vi "日志、报警信息存储 (子VI).vi"() -> ()   [LabVIEW 2016, in "德润DR803F超标留样.lvlib"]
panel:
  out "仪器状态":T1 {"门状态" items=["关闭", "打开"]; "采样模式" items=["定时留样"=1, "时间等比"=2, "同步留样"=3, "外控留样"=4, "超标留样"=5]; "工作进程" items=["清洗管路初始化", "采样瓶位置初始化", "采样瓶排空", "清洗管下降", "采样瓶清洗", "清洗管上升", "外置泵延时", "管路润洗", "进样1", "进样2", "排空管路", "采样瓶位置调整", "待机"]; "仪器时间" format="%<%Y/%m/%d %H:%M:%S>T"; "工作状态" items=["停止", "运行"]}
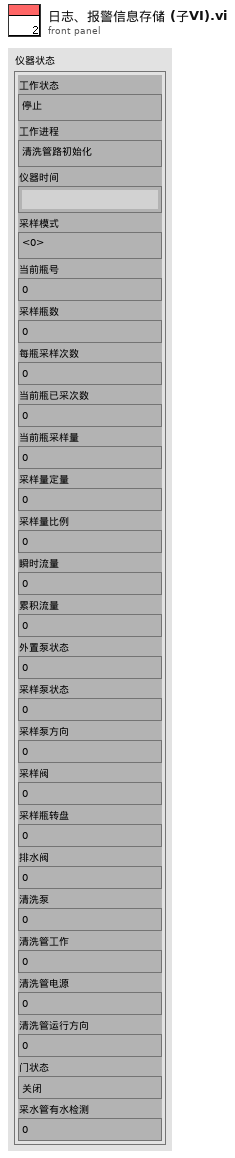
[diagram p1: front panel]
types:
  T1 = cluster{"工作状态":u16, "工作进程":u16, "仪器时间":timestamp, "采样模式":u16, "当前瓶号":dbl, "采样瓶数":dbl, "每瓶采样次数":dbl, "当前瓶已采次数":dbl, "当前瓶采样量":dbl, "采样量定量":dbl, "采样量比例":dbl, "瞬时流量":dbl, "累积流量":dbl, "外置泵状态":dbl, "采样泵状态":dbl, "采样泵方向":dbl, "采样阀":dbl, "采样瓶转盘":dbl, "排水阀":dbl, "清洗泵":dbl, "清洗管工作":dbl, "清洗管电源":dbl, "清洗管运行方向":dbl, "门状态":u16, "采水管有水检测":dbl}
  T2 = cluster{"时间标识":timestamp, "设备":string, "日志信息":string, "流程参数":string}
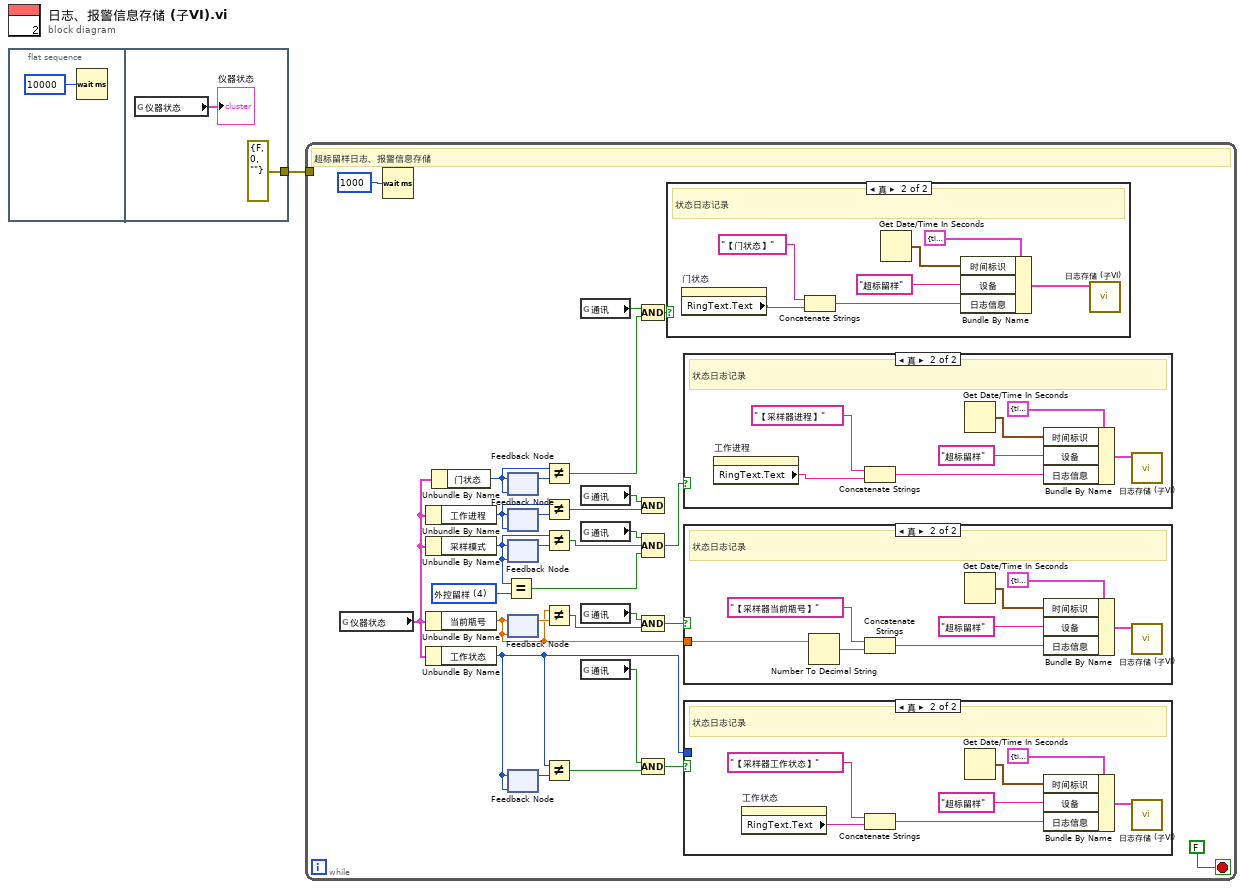
[diagram p0: block diagram]
diagram:
  n1 = flat-sequence {
    tunnel: [errorcluster {"status"=FALSE, "code"=0, "source"=""} ("错误常量")] -> w1
    frame #0 {
      n2 = Wait (ms)(milliseconds to wait=u32 10000 ("等待时间（毫秒）")) -> ()  [unwired: 1 out]
    }
    frame #1 {
      n3 = global read "超标留样全局.vi" "仪器状态"() -> (→"仪器状态":T1)
    }
  }
  n4 = while {
    tunnel: w1 -> [_]
    stop <- FALSE stop-if-true
    w6 = u16 4 items=["定时留样"=1, "时间等比"=2, "同步留样"=3, "外控留样"=4, "超标留样"=5] ("采样模式")
    # "超标留样日志、报警信息存储"
    n5 = global read "超标留样全局.vi" "仪器状态"() -> (w7:T1)
    n6 = Wait (ms)(milliseconds to wait=u32 1000 ("等待时间（毫秒）")) -> ()  [unwired: 1 out]
    n7 = Unbundle By Name(w7) -> ("工作进程"=w31:u16)
    n8 = Unbundle By Name(w7) -> ("采样模式"=w23:u16)
    n9 = Unbundle By Name(w7) -> ("当前瓶号"=w28:dbl)
    n10 = Unbundle By Name(w7) -> ("工作状态"=w27:u16)
    n11 = Unbundle By Name(w7) -> ("门状态"=w24:u16)
    n12 = Equal?(x=w23, y=w6) -> (x = y?=w9:bool)
    n13 = feedback #1(w24) -> (w25:u16)
    n14 = feedback-in #1(w24) -> ()
    n15 = feedback #2(w31) -> (w30:u16)
    n16 = feedback-in #2(w31) -> ()
    n17 = feedback #3(w23) -> (w22:u16)
    n18 = feedback-in #3(w23) -> ()
    n19 = feedback #4(w28) -> (w29:dbl)
    n20 = feedback-in #4(w28) -> ()
    n21 = feedback #5(w27) -> (w26:u16)
    n22 = feedback-in #5(w27) -> ()
    n23 = Not Equal?(x=w24, y=w25) -> (x != y?=w19:bool)
    n24 = Not Equal?(x=w31, y=w30) -> (x != y?=w17:bool)
    n25 = Not Equal?(x=w23, y=w22) -> (x != y?=w8:bool)
    n26 = Not Equal?(x=w28, y=w29) -> (x != y?=w14:bool)
    n27 = Not Equal?(x=w27, y=w26) -> (x != y?=w12:bool)
    n28 = global read "超标留样全局.vi" "通讯"() -> (w21:bool)
    n29 = global read "超标留样全局.vi" "通讯"() -> (w18:bool)
    n30 = global read "超标留样全局.vi" "通讯"() -> (w10:bool)
    n31 = global read "超标留样全局.vi" "通讯"() -> (w16:bool)
    n32 = global read "超标留样全局.vi" "通讯"() -> (w13:bool)
    n33 = Compound Arithmetic op=AND ("复合运算")(w21, w19) -> (w20:bool)
    n34 = Compound Arithmetic op=AND ("复合运算")(w18, w17) -> ()  [unwired: 1 out]
    n35 = Compound Arithmetic op=AND ("复合运算")(w10, w8, w9) -> (w5:bool)
    n36 = Compound Arithmetic op=AND ("复合运算")(w16, w14) -> (w15:bool)
    n37 = Compound Arithmetic op=AND ("复合运算")(w13, w12) -> (w11:bool)
    n38 = case shown="真" w20 {
      frame False {
      }
      frame True {
        # "状态日志记录"
        n39 = property on="门状态" class="Ring (严格)"() -> ("RingText.Text"=w34:string)  [unwired: 2 in, 2 out]
        n40 = Concatenate Strings("【门状态】" ("日志信息"), w34) -> (w40:string)
        n41 = Get Date/Time In Seconds() -> (seconds since 1Jan1904=w37:timestamp)
        n42 = Bundle By Name(cluster=T2 {"时间标识"=timestamp(0 s since 1904-01-01), "设备"="", "日志信息"="", "流程参数"=""} ("data in"), "时间标识"=w37, "设备"="超标留样", "日志信息"=w40) -> (w36:T2)
        n43 = call "日志存储 (子VI).vi"("data in"=w36) -> ()  [unwired: 11 in]
      }
    }
    n44 = case shown="真" w5 {
      frame False {
      }
      frame True {
        # "状态日志记录"
        n45 = property on="工作进程" class="Ring (严格)"() -> ("RingText.Text"=w56:string)  [unwired: 2 in, 2 out]
        n46 = Concatenate Strings("【采样器进程】" ("日志信息"), w56) -> (w62:string)
        n47 = Get Date/Time In Seconds() -> (seconds since 1Jan1904=w59:timestamp)
        n48 = Bundle By Name(cluster=T2 {"时间标识"=timestamp(0 s since 1904-01-01), "设备"="", "日志信息"="", "流程参数"=""} ("data in"), "时间标识"=w59, "设备"="超标留样", "日志信息"=w62) -> (w58:T2)
        n49 = call "日志存储 (子VI).vi"("data in"=w58) -> ()  [unwired: 11 in]
      }
    }
    n50 = case shown="真" w15 {
      tunnel: w28 -> [_ w49]
      frame False {
      }
      frame True {
        # "状态日志记录"
        n51 = Number To Decimal String(number=w49) -> (decimal integer string=w48:string)  [unwired: 1 in]
        n52 = Concatenate Strings("【采样器当前瓶号】" ("日志信息"), w48) -> (w55:string)
        n53 = Get Date/Time In Seconds() -> (seconds since 1Jan1904=w52:timestamp)
        n54 = Bundle By Name(cluster=T2 {"时间标识"=timestamp(0 s since 1904-01-01), "设备"="", "日志信息"="", "流程参数"=""} ("data in"), "时间标识"=w52, "设备"="超标留样", "日志信息"=w55) -> (w51:T2)
        n55 = call "日志存储 (子VI).vi"("data in"=w51) -> ()  [unwired: 11 in]
      }
    }
    n56 = case shown="真" w11 {
      tunnel: w27 -> [_ _]
      frame False {
      }
      frame True {
        # "状态日志记录"
        n57 = property on="工作状态" class="Ring (严格)"() -> ("RingText.Text"=w41:string)  [unwired: 2 in, 2 out]
        n58 = Concatenate Strings("【采样器工作状态】" ("日志信息"), w41) -> (w47:string)
        n59 = Get Date/Time In Seconds() -> (seconds since 1Jan1904=w44:timestamp)
        n60 = Bundle By Name(cluster=T2 {"时间标识"=timestamp(0 s since 1904-01-01), "设备"="", "日志信息"="", "流程参数"=""} ("data in"), "时间标识"=w44, "设备"="超标留样", "日志信息"=w47) -> (w43:T2)
        n61 = call "日志存储 (子VI).vi"("data in"=w43) -> ()  [unwired: 11 in]
      }
    }
  }
